vi "Variables Read for Tension Control.vi"() -> (2 "Manual Control?":bool, 3 "Manual Control":dbl[](array[numeric]), 4 "Tension Control On":bool, 5 "Motor Enable":bool[](array[boolean]), 7 "Encoder Initialize":bool)   [LabVIEW 2021]
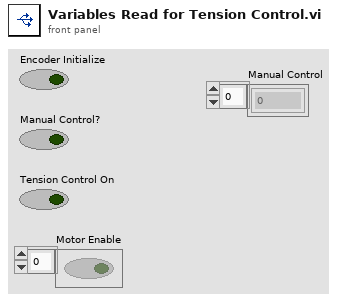
[diagram p1: front panel]
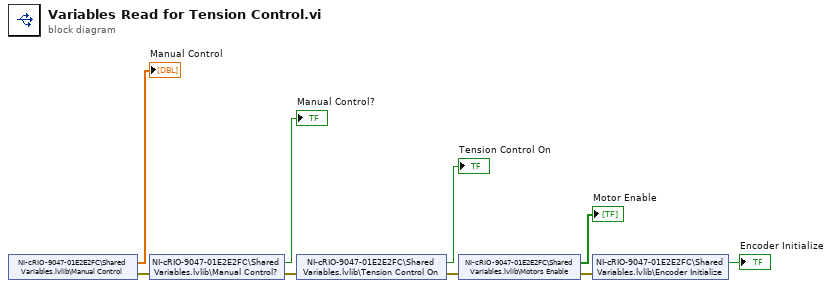
[diagram p0: block diagram]
diagram:
  n1 = shared-variable "NI-cRIO-9047-01E2E2FC\\Shared Variables.lvlib\\Manual Control"() -> (→"Manual Control":dbl[], error out=w4:errorcluster)  [unwired: 1 in]
  n2 = shared-variable "NI-cRIO-9047-01E2E2FC\\Shared Variables.lvlib\\Manual Control?"(error in=w4) -> (→"Manual Control?":bool, error out=w3:errorcluster)
  n3 = shared-variable "NI-cRIO-9047-01E2E2FC\\Shared Variables.lvlib\\Tension Control On"(error in=w3) -> (→"Tension Control On":bool, error out=w2:errorcluster)
  n4 = shared-variable "NI-cRIO-9047-01E2E2FC\\Shared Variables.lvlib\\Motors Enable"(error in=w2) -> (→"Motor Enable":bool[], error out=w1:errorcluster)
  n5 = shared-variable "NI-cRIO-9047-01E2E2FC\\Shared Variables.lvlib\\Encoder Initialize"(error in=w1) -> (→"Encoder Initialize":bool)  [unwired: 1 out]
